vi "Read.vi"(7 "Max Data Length":i32=1024, 8 "Error In":errorcluster, 11 "SFTP File In":refnum<class "SFTP File.lvclass">) -> (0 "Error Out":errorcluster, 1 "End-of-File?":bool, 2 "Data":u8[](array[numeric]), 3 "SFTP File Out":refnum<class "SFTP File.lvclass">)   [LabVIEW 2017, in "Toolkit.lvlib" / "SFTP File.lvclass"]
uses:
  SFTP File.lvclass
  SFTP File.lvclass/SFTP File.ctl
  Toolkit.lvlib
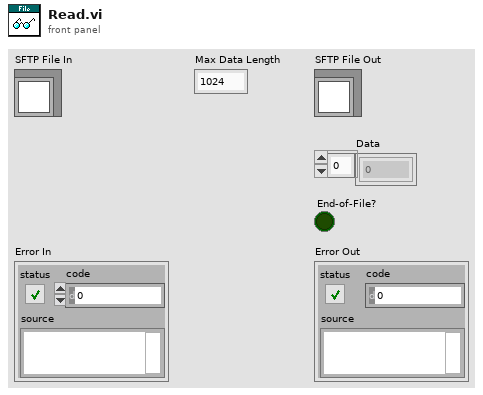
[diagram p1: front panel]
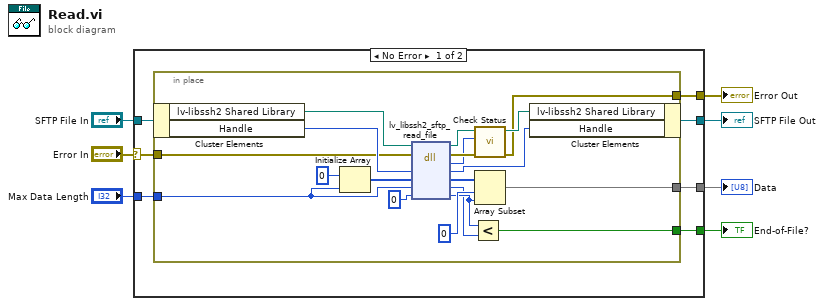
[diagram p0: block diagram]
diagram:
  n1 = case shown="No Error" "Error In" {
    selector: "Error In" -> [w13 w34]
    tunnel: "SFTP File In" -> [w14 w35]
    tunnel: [w12 w35] -> w4
    tunnel: [w11 w34] -> w5
    tunnel: [w10 _] -> w3
    tunnel: "Max Data Length" -> [w9 _]
    tunnel: [w8 _] -> w1
    frame No Error {
      n2 = in-place {
        in-place-border: w13 -> [w31]
        in-place-border: [w25] -> w11
        in-place-border: [w18] -> w10
        in-place-border: w9 -> [w22]
        in-place-border: [w15] -> w8
        n3 = in-place-cluster #1(w14) -> ("lv-libssh2 Shared Library"=w33:path, "Handle"=w32:u64)
        n4 = Initialize Array(u8 0, w22) -> (w23:u8[])
        n5 = dll-call lib="D:/Users/cfield/Code/Field R&D Services/SSH/LV-LIBSSH2/LabVIEW/trunk/src/Toolkit/Support/lv-libssh2.*" fn="lv_libssh2_sftp_read_file"(path in=w33, error in=w31, "handle"=w32, "buffer"=w23, "buffer_max_length"=w22, "read_count"=i64 0) -> (path out=w28:path, error out=w29:errorcluster, "status"=w26:i32, "handle"=w30:u64, "buffer"=w20:u8[], "buffer_max_length"=w16:u64, "read_count"=w17:i64)  [unwired: 1 in]
        n6 = Less?(x=w17, y=w16) -> (x < y?=w15:bool)
        n7 = call "Check Status.vi"("Error In"=w29, "Status"=w26, "lv-libssh2 Shared Library In"=w28) -> ("Error Out"=w25:errorcluster, "lv-libssh2 Shared Library Out"=w27:path)  [unwired: 7 in]
        n8 = Array Subset(array=w20, index=0, length=w17) -> (w18:u8[])
        n9 = in-place-cluster #1("lv-libssh2 Shared Library"=w27, "Handle"=w30) -> (w12:refnum<class "SFTP File.lvclass">)
      }
    }
    frame Error {
    }
  }
  "Error Out" <- w5
  "SFTP File Out" <- w4
  "Data" <- w3
  "End-of-File?" <- w1
